vi "Unit Vector.vi"   [LabVIEW 2012, in "NI_AALBase.lvlib"]
doc: "Finds the <B>norm</B> of the <B>Input Vector</B> and obtains its corresponding <B>Unit Vector</B> by normalizing the original <B>Input Vector</B> with its <B>norm</B>."
uses:
  NI_AALBase.lvlib
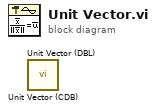
[diagram p0: block diagram]
diagram:
  n1 = call "Unit Vector (CDB).vi"() -> ()  [unwired: 9 in, 3 out]
  n2 = call "Unit Vector (DBL).vi"() -> ()  [unwired: 9 in, 3 out]
